vi "闹钟（分）.vi"(5 "设置分":i32=5, 7 "启用":bool=TRUE) -> (6 "时间到脉冲":bool, 8 "分":i32)   [LabVIEW 2012]
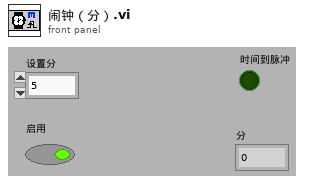
[diagram p1: front panel]
types:
  T1 = typedef "LVDateTimeRec.ctl" = cluster{"秒数的小数部分":dbl, "秒":i32, "分":i32, "时":i32, "日":i32, "月":i32, "年":i32, "天数（周）":i32, "天数（年）":i32, "DST":i32}
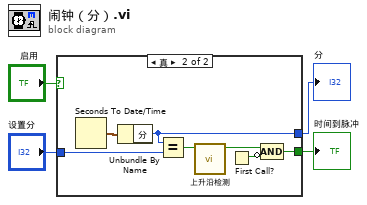
[diagram p0: block diagram]
diagram:
  n1 = case shown="真" "启用" {
    tunnel: [_ w8] -> w4
    tunnel: "设置分" -> [_ w7]
    tunnel: [_ w10] -> w1
    frame False {
    }
    frame True {
      n2 = Seconds To Date/Time() -> (date time rec=w11:T1)  [unwired: 2 in]
      n3 = Unbundle By Name(w11) -> ("分"=w8:i32)
      n4 = Equal?(x=w8, y=w7) -> (x = y?=w6:bool)
      n5 = call "上升沿检测.vi"("input"=w6) -> ("output"=w5:bool)  [unwired: 9 in, 1 out]
      n6 = First Call?() -> (First Call?: T/F=w9:bool)
      n7 = Compound Arithmetic op=AND(w5, invert w9) -> (w10:bool)
    }
  }
  "时间到脉冲" <- w1
  "分" <- w4
